vi "Remove_Duplicates_1D.vi"(10 "Input Array":dbl[](array[numeric])) -> (1 "Unique Array":dbl[](array[numeric]), 3 "Removed indicies":i32[](array[numeric]))   [LabVIEW 2011]
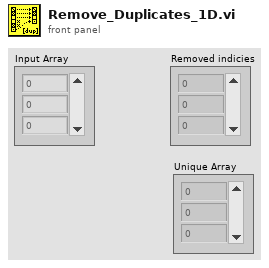
[diagram p1: front panel]
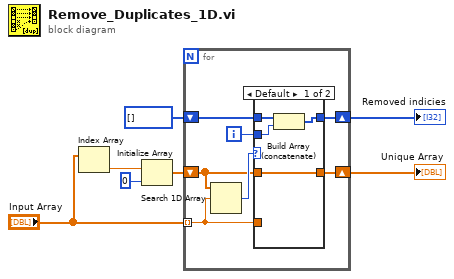
[diagram p0: block diagram]
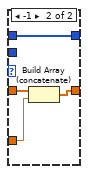
[diagram p2: hidden frame]
diagram:
  n1 = Index Array(array="Input Array") -> (element=w5:dbl)  [unwired: 1 in]
  n2 = Initialize Array(w5, 0 ("Dimension Size")) -> (w6:dbl[])
  n3 = for {
    tunnel: "Input Array" -> [w13] mode=indexing
    shift-right: [w12] -> w1
    shift-left: w6 -> [w11]
    shift-right: [w9] -> w3
    shift-left: i32[] [] -> [w8]
    i -> [w10]
    n4 = Search 1D Array(1D array=w11, element=w13) -> (index of element=w14:i32)  [unwired: 1 in]
    n5 = case shown="Default" w14 {
      tunnel: w13 -> [_ w22]
      tunnel: [w18 w20] -> w12
      tunnel: w11 -> [w18 w21]
      tunnel: w10 -> [w15 _]
      tunnel: [w16 w19] -> w9
      tunnel: w8 -> [w17 w19]
      frame Default {
        n6 = Build Array (concatenate)(w17, w15) -> (w16:i32[])
      }
      frame -1 {
        n7 = Build Array (concatenate)(w21, w22) -> (w20:dbl[])
      }
    }
  }
  "Removed indicies" <- w3
  "Unique Array" <- w1
